vi "BRig_Host__Loop_Consumer_RunState__closeLoop_getData_dataPlot.vi"(10 "input_idx":i32[](array[numeric]), 11 "input_dataPlot":u16[][](array[numeric])) -> (3 "output_dataPlot":u16[][](array[numeric]))   [LabVIEW 2014]
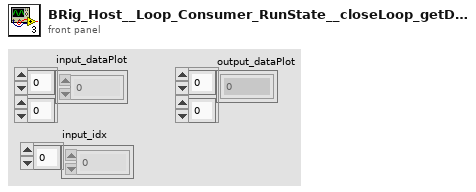
[diagram p1: front panel]
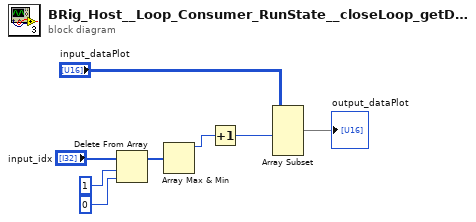
[diagram p0: block diagram]
diagram:
  n1 = Delete From Array(array="input_idx", length=1, index=0) -> (array with subset deleted=w3:i32[])  [unwired: 1 out]
  n2 = Array Max & Min(array=w3) -> (max value=w2:i32)  [unwired: 3 out]
  n3 = Increment(x=w2) -> (x+1=w1:i32)
  n4 = Array Subset(array="input_dataPlot", length (row)=w1) -> (→"output_dataPlot":u16[][])  [unwired: 3 in]
